vi "Robot Velocity to LR.vi"(8 "Trackwidth":dbl=30.0 format="%#_13g", 9 "Max Accel":dbl, 10 "Max Velocity":dbl, 11 "Curvature":dbl) -> (2 "r":dbl, 3 "l":dbl)   [LabVIEW 2019, in "Pure Pursuit.lvlib"]
uses:
  Pure Pursuit.lvlib
  Typedef/Path AE Action.ctl
  <vilib>/addons/control/pid/pid.llb/PID Output Rate Limiter (DBL).vi
  <vilib>/addons/control/pid/NI_PID_pid.lvlib
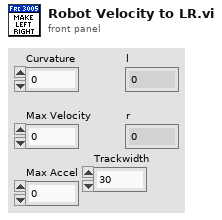
[diagram p1: front panel]
types:
  T1 = typedef "Pure Pursuit.lvlib/Path AE Action.ctl" = enum16{"Initialize", "Get Close Point", "Get Target Point", "Default", "Get Point", "Get Distance Remaining"}
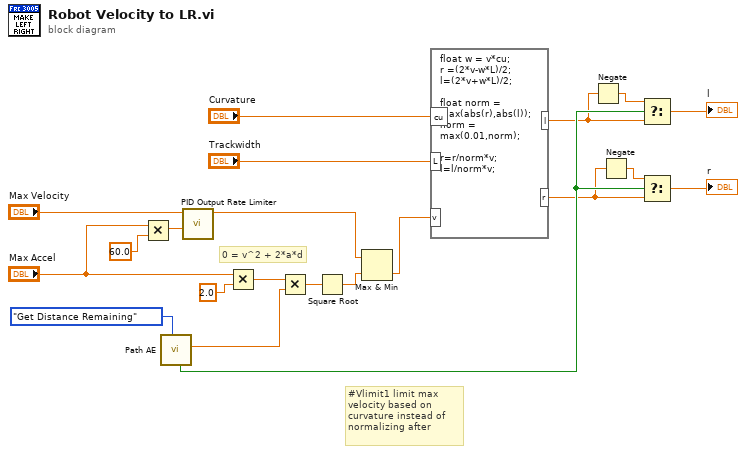
[diagram p0: block diagram]
diagram:
  # "0 = v^2 + 2*a*d"
  # "#Vlimit1 limit max velocity based on curvature instead of normalizing after"
  n1 = Multiply(x="Max Accel", y=60.0) -> (x*y=w10:dbl)
  n2 = call "Path AE.vi"("Path AE Action"=Path_AE_Action."Get Distance Remaining") -> ("Distance"=w15:dbl, "Reverse? (F)"=w5:bool)  [unwired: 5 in, 4 out]
  n3 = call-poly <vilib>:"PID Output Rate Limiter.vi"("output rate (EGU/min)"=w10, "input (controller output)"="Max Velocity") -> ("output"=w12:dbl)  [unwired: 6 in, 1 out]
  n4 = Multiply(x="Max Accel", y=2.0) -> (x*y=w16:dbl)
  n5 = Multiply(x=w16, y=w15) -> (x*y=w14:dbl)
  n6 = Square Root(x=w14) -> (sqrt(x)=w13:dbl)
  n7 = Max & Min(x=w12, y=w13) -> (min(x,y)=w11:dbl)  [unwired: 1 out]
  n8 = formula code="float w = v*cu;\nr =(2*v-w*L)/2;\nl=(2*v+w*L)/2;\n\nfloat norm = max(abs(r),abs(l));\nnorm = max(0.01,norm);\n\nr=r/norm*v;\nl=l/norm*v;"("L"="Trackwidth", "cu"="Curvature", "v"=w11) -> ("r"=w2:dbl, "l"=w1:dbl)
  n9 = Negate(x=w1) -> (-x=w4:dbl)
  n10 = Negate(x=w2) -> (-x=w3:dbl)
  n11 = Select(t=w4, s=w5, f=w1) -> (s? t:f=→"l":dbl)
  n12 = Select(t=w3, s=w5, f=w2) -> (s? t:f=→"r":dbl)
